vi "graph temp.vi"() -> ()   [LabVIEW 2014]
uses:
  Instance           4 18Saved   graph temp .vi
panel:
  out "temp 2":ext[](array[numeric]) format="%#_10e"
  out "R(temp) 2":ext(graph)
  in  "Mult Temp baño 2":u16(ring)=1 items=["3458", "34420", "34401"]
  in  "addrss instr 2  (board addrs:instrum addrs) 2":string="0:13"
  out "adrs temp baño \n(board addrs:instrum addrs) 2":string="0:6"
  in  "addrss instr 1  (board addrs:instrum addrs)":string="0:14"
  out "R(temp)":ext(graph)
  out "temp":ext[](array[numeric]) format="%#_10e"
  in  "File Name":path=path "F:/gonzalo/Mediciones"
  in  "stop":bool
  out "adrs temp baño \n(board addrs:instrum addrs)":string="0:6"
  in  "Mult Temp baño":u16(ring)=2 items=["3458", "34420", "34401"]
  # "Instrucciones\n1- seleccionar directorio y file name\n2- seleccione multimetro a utilizar y addrss\n2- play empieza a graficar y grabar medidas\n3- stop, finaliza (mantener apretado)"
  # "MEDICION TEMP CON 3458"
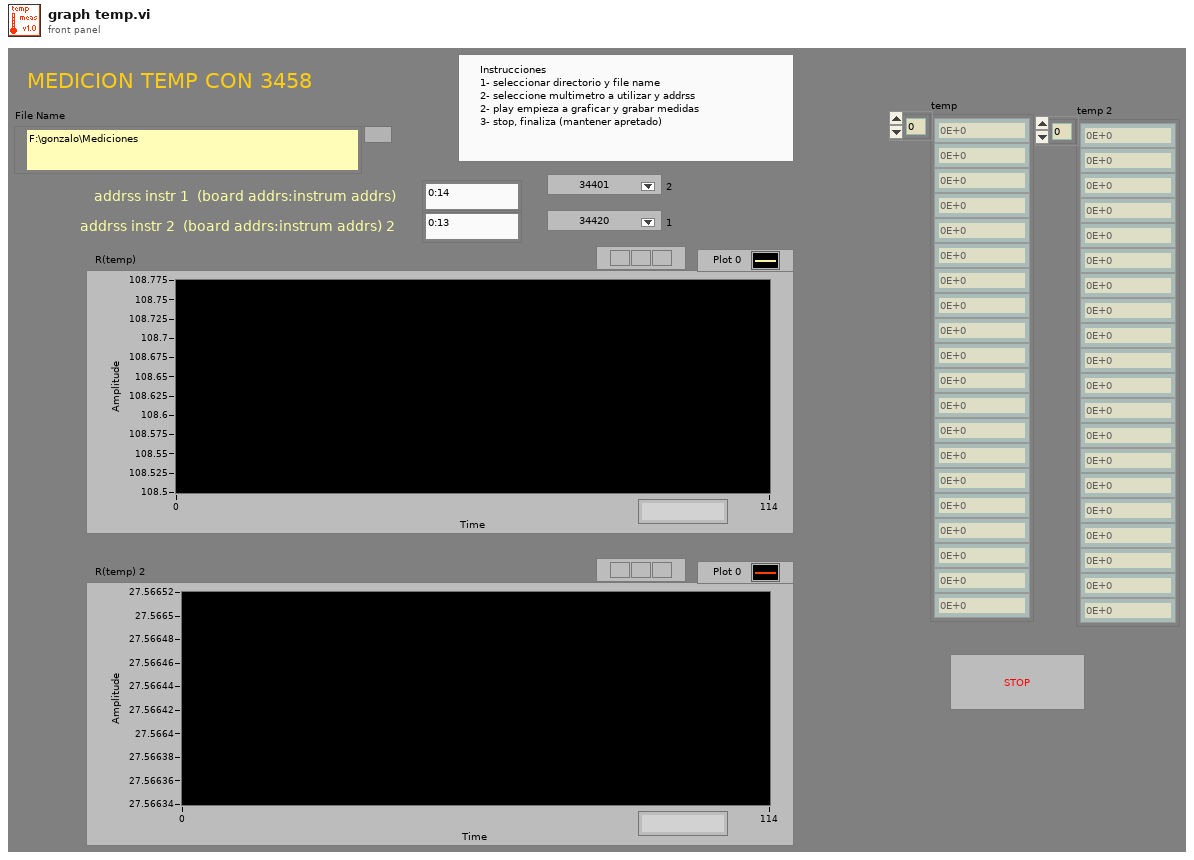
[diagram p1: front panel]
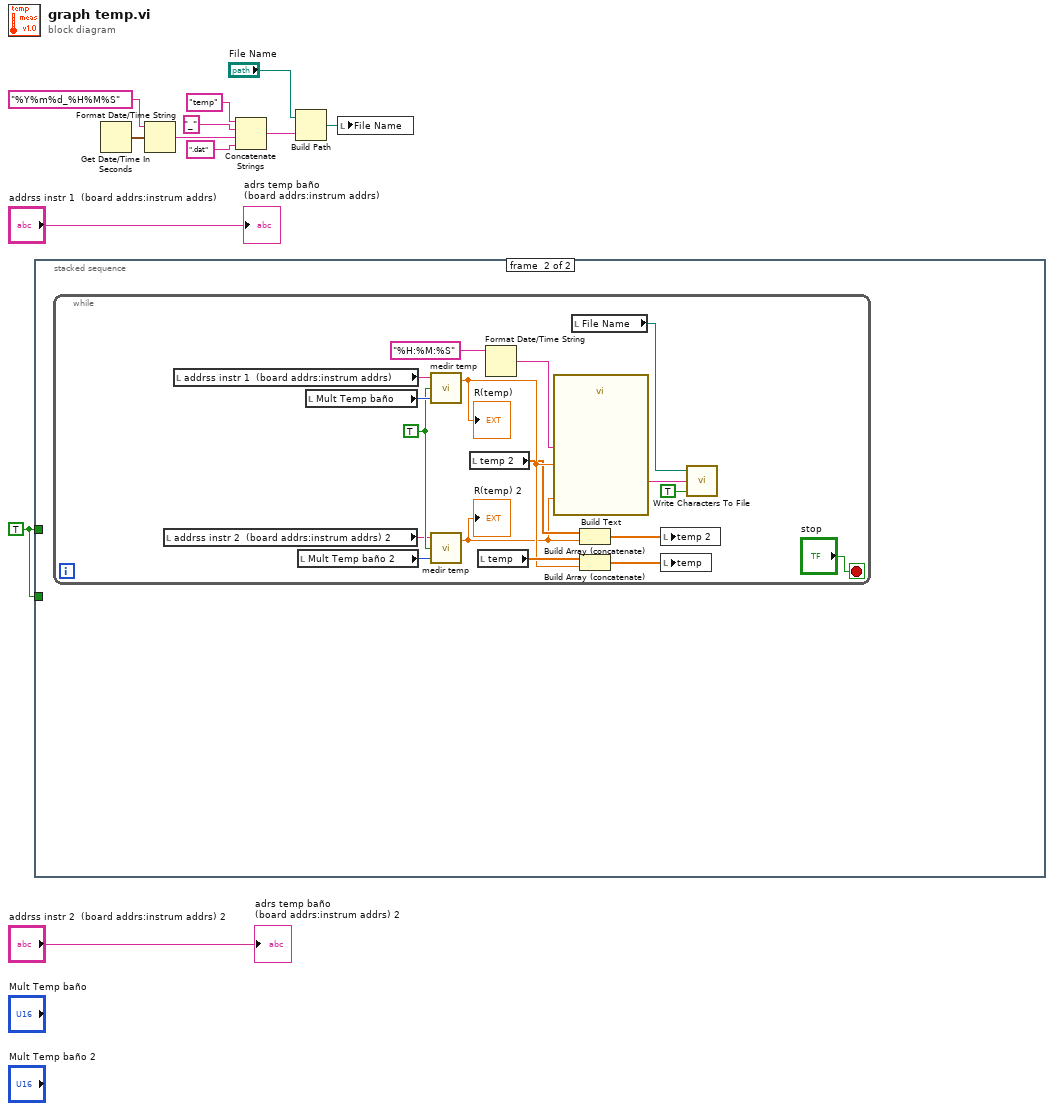
[diagram p0: block diagram]
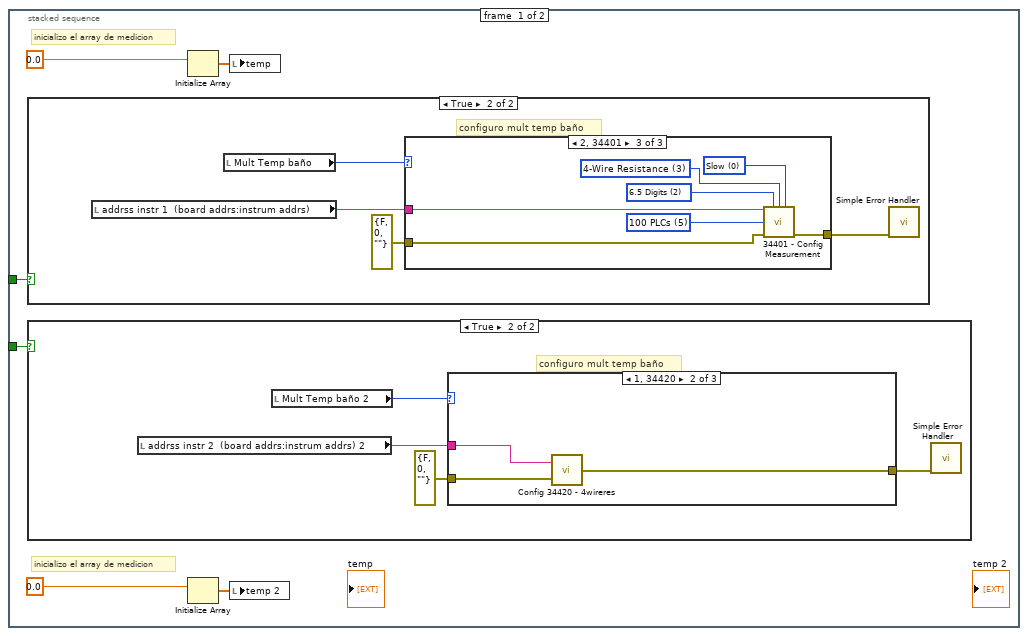
[diagram p2: hidden frame]
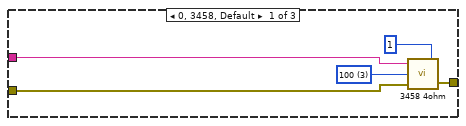
[diagram p4: hidden frame]
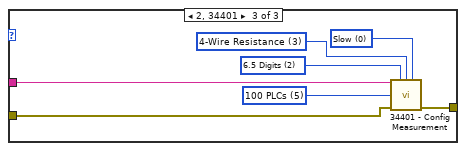
[diagram p5: hidden frame]
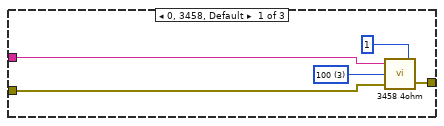
[diagram p7: hidden frame]
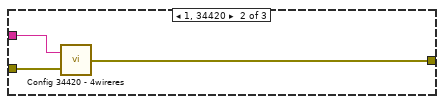
[diagram p8: hidden frame]
diagram:
  w1 = TRUE
  n1 = stacked-sequence {
    tunnel: w1 -> [w16 _]
    tunnel: w1 -> [w15 _]
    frame #0 {
      # "inicializo el array de medicion"
      # "inicializo el array de medicion"
      n2 = case shown="True" w16 {
        frame False {
        }
        frame True {
          # "configuro mult temp baño"
          n3 = local read "addrss instr 1  (board addrs:instrum addrs)"() -> (w40:string)
          n4 = local read "Mult Temp baño"() -> (w41:u16)
          n5 = case shown="2, 34401" w41 {
            tunnel: w40 -> [w45 w49 w52]
            tunnel: errorcluster {"status"=FALSE, "code"=0, "source"=""} ("error OUT 2") -> [w46 w48 w51]
            tunnel: [w42 w47 w50] -> w38
            frame 0, 3458, Default {
              w43 = u16 3 items=["10", "20", "50", "100", "200"] ("NPLC")
              n6 = call "3458 4ohm.vi"("NRDGS"=1, "error in (no error)"=w46, "NPLC"=w43, "Multímetro TRP"=w45) -> ("error out"=w42:errorcluster)
            }
            frame 1, 34420 {
              n7 = call "Config 34420 - 4wireres.vi"("error IN"=w48, "Address 34420 (default: 13)"=w49) -> ("error out"=w47:errorcluster)
            }
            frame 2, 34401 {
              w56 = u16 5 items=["Default", "0.02 PLCs", "0.2 PLC", "1 PLCs", "10 PLCs", "100 PLCs"] ("Manual Int. (0:Default)")
              w55 = u16 0 items=["Slow", "Medium", "Fast"] ("AC Filter (1:Medium)")
              w54 = u16 3 items=["DC Voltage", "AC Voltage", "2--Wire Resistance", "4-Wire Resistance", "DC Current", "AC Current", "Frequency", "Period", "Continuity", "Diode Checking", "VDC: VDC Ratio"] ("Function (0:V DC)")
              w53 = u16 2 items=["4.5 Digits", "5.5 Digits", "6.5 Digits"] ("Manual Res. (1:5.5 Digits)")
              n8 = call "34401 - Config Measurement.vi"("address"=w52, "Manual Res. (1:5.5 Digits)"=w53, "Function (0:V DC)"=w54, "AC Filter (1:Medium)"=w55, "Manual Int. (0:Default)"=w56, "error in (no error)"=w51) -> ("error out"=w50:errorcluster)  [unwired: 9 in]
            }
          }
          n9 = call <vilib>:"Simple Error Handler.vi"("error in (no error)"=w38) -> ()  [unwired: 4 in, 5 out]
        }
      }
      n10 = case shown="True" w15 {
        frame False {
        }
        frame True {
          # "configuro mult temp baño"
          n11 = local read "addrss instr 2  (board addrs:instrum addrs) 2"() -> (w21:string)
          n12 = local read "Mult Temp baño 2"() -> (w22:u16)
          n13 = case shown="1, 34420" w22 {
            tunnel: w21 -> [w26 w30 w33]
            tunnel: errorcluster {"status"=FALSE, "code"=0, "source"=""} ("error OUT 2") -> [w27 w29 w32]
            tunnel: [w23 w28 w31] -> w19
            frame 0, 3458, Default {
              w24 = u16 3 items=["10", "20", "50", "100", "200"] ("NPLC")
              n14 = call "3458 4ohm.vi"("NRDGS"=1, "error in (no error)"=w27, "NPLC"=w24, "Multímetro TRP"=w26) -> ("error out"=w23:errorcluster)
            }
            frame 1, 34420 {
              n15 = call "Config 34420 - 4wireres.vi"("error IN"=w29, "Address 34420 (default: 13)"=w30) -> ("error out"=w28:errorcluster)
            }
            frame 2, 34401 {
              w37 = u16 5 items=["Default", "0.02 PLCs", "0.2 PLC", "1 PLCs", "10 PLCs", "100 PLCs"] ("Manual Int. (0:Default)")
              w36 = u16 0 items=["Slow", "Medium", "Fast"] ("AC Filter (1:Medium)")
              w35 = u16 3 items=["DC Voltage", "AC Voltage", "2--Wire Resistance", "4-Wire Resistance", "DC Current", "AC Current", "Frequency", "Period", "Continuity", "Diode Checking", "VDC: VDC Ratio"] ("Function (0:V DC)")
              w34 = u16 2 items=["4.5 Digits", "5.5 Digits", "6.5 Digits"] ("Manual Res. (1:5.5 Digits)")
              n16 = call "34401 - Config Measurement.vi"("address"=w33, "Manual Res. (1:5.5 Digits)"=w34, "Function (0:V DC)"=w35, "AC Filter (1:Medium)"=w36, "Manual Int. (0:Default)"=w37, "error in (no error)"=w32) -> ("error out"=w31:errorcluster)  [unwired: 9 in]
            }
          }
          n17 = call <vilib>:"Simple Error Handler.vi"("error in (no error)"=w19) -> ()  [unwired: 4 in, 5 out]
        }
      }
      n18 = Initialize Array(0.0 ("element")) -> (w17:dbl[])  [unwired: 1 in]
      n19 = Initialize Array(0.0 ("element")) -> (w14:dbl[])  [unwired: 1 in]
      n20 = local write "temp"(w17) -> ()
      n21 = local write "temp 2"(w14) -> ()
    }
    frame #1 {
      n22 = while {
        stop <- "stop" stop-if-true
        w60 = TRUE ("Medir Temperatura")
        n23 = local read "addrss instr 2  (board addrs:instrum addrs) 2"() -> (w59:string)
        n24 = local read "addrss instr 1  (board addrs:instrum addrs)"() -> (w72:string)
        n25 = local read "Mult Temp baño 2"() -> (w58:u16)
        n26 = local read "Mult Temp baño"() -> (w73:u16)
        n27 = call "medir temp.vi"("multimetro"=w73, "Medir Temperatura"=w60, "address string"=w72) -> ("Numeric"=w64:ext)  [unwired: 1 in]
        "R(temp)" <- w64
        n28 = call "medir temp.vi"("multimetro"=w58, "Medir Temperatura"=w60, "address string"=w59) -> ("Numeric"=w57:ext)  [unwired: 1 in]
        "R(temp) 2" <- w57
        n29 = local read "temp 2"() -> (w62:ext[])
        n30 = local read "temp"() -> (w67:ext[])
        n31 = Format Date/Time String(time format string (%c)="%H:%M:%S") -> (date/time string=w68:string)  [unwired: 2 in]
        n32 = call "Build Text"("tiempo"=w68, "Temp Multimetro 1"=w64, "Temp Multimetro 2"=w57) -> ("Result"=w70:string)  [unwired: 11 in, 1 out]
        n33 = local read "File Name"() -> (w63:path)
        n34 = Build Array (concatenate)(w62, w57) -> (w61:ext[])
        n35 = Build Array (concatenate)(w67, w64) -> (w65:ext[])
        n36 = local write "temp 2"(w61) -> ()
        n37 = local write "temp"(w65) -> ()
        n38 = call <vilib>:"Write Characters To File.vi"("append to file? (new file:F)"=TRUE, "character string"=w70, "file path (dialog if empty)"=w63) -> ()  [unwired: 2 in, 1 out]
      }
    }
  }
  n39 = Get Date/Time In Seconds() -> (seconds since 1Jan1904=w5:timestamp)
  n40 = Format Date/Time String(time format string (%c)="%Y%m%d_%H%M%S", seconds (now)=w5) -> (date/time string=w3:string)  [unwired: 1 in]
  n41 = Concatenate Strings("temp" ("string"), "_" ("string"), w3, ".dat" ("string")) -> (w7:string)
  n42 = Build Path(base path="File Name", name or relative path=w7) -> (appended path=w6:path)
  n43 = local write "File Name"(w6) -> ()
  "adrs temp baño \n(board addrs:instrum addrs)" <- "addrss instr 1  (board addrs:instrum addrs)"
  "adrs temp baño \n(board addrs:instrum addrs) 2" <- "addrss instr 2  (board addrs:instrum addrs) 2"
